vi "Create_Pos_array.vi"(2 "Traverse line":T1 {"Row Duration (mins)" format="%#.1f"; "Row No" min=0; "Trace Gas Concentration (%)" min=0.0 format="%#.2f"; "Emission Rate (l/min)" format="%#.2f"; "Tunnel Speed" format="%#.2f"; "Start X" format="%#.2f"; "Start Y" format="%#.2f"; "Start Z" format="%#.2f"; "End X" format="%#.2f"; "End Y" format="%#.2f"; "End Z" format="%#.2f"; "Averaging time (min)" min=0.0 format="%#.2f"}) -> (5 "Traverse line Out":T1 {"Row Duration (mins)" format="%#.1f"; "Row No" min=0; "Trace Gas Concentration (%)" min=0.0 format="%#.2f"; "Emission Rate (l/min)" format="%#.2f"; "Tunnel Speed" format="%#.2f"; "Start X" format="%#.2f"; "Start Y" format="%#.2f"; "Start Z" format="%#.2f"; "End X" format="%#.2f"; "End Y" format="%#.2f"; "End Z" format="%#.2f"; "Averaging time (min)" min=0.0 format="%#.2f"}, 6 "Error Messages":string, 7 "Array of Positions":dbl[][](array[numeric]) format="%.2f", 9 "Axis Traversed":enum16{"X traverse", "Y traverse", "Z traverse"}(ring))   [LabVIEW 2012]
uses:
  Traverse_cluster.ctl
  Spacing.ctl
  Controls/Multi_run_mode.ctl
  Globals/Extra_Commands_Global.vi
panel:
  # "X           Y            Z"
  # "Start"
  # "End"
  # "X           Y            Z"
  # "Start"
  # "End"
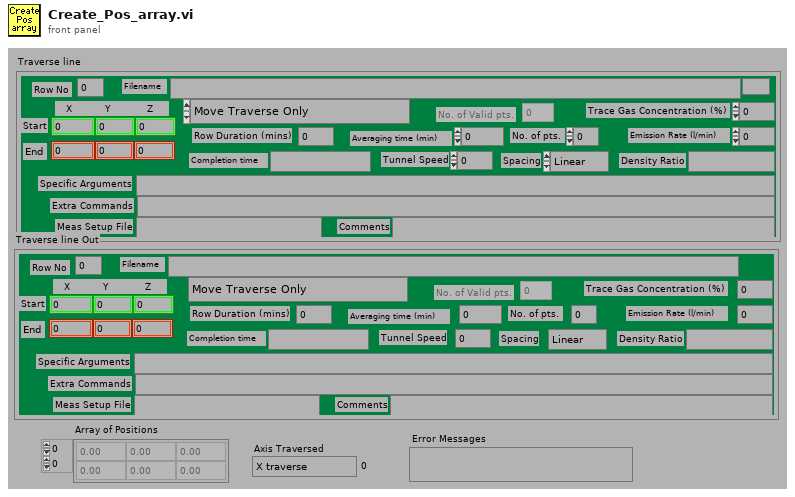
[diagram p1: front panel]
types:
  T1 = typedef "Traverse_cluster.ctl" = cluster{"Start X":dbl, "Start Y":dbl, "Start Z":dbl, "End X":dbl, "End Y":dbl, "End Z":dbl, "No. of pts.":i32, "Spacing":T2, "Filename":path, "Tunnel Speed":dbl, "Averaging time (min)":dbl, "Extra Commands":string, "Specific Arguments":string, "Emission Rate (l/min)":dbl, "Trace Gas Concentration (%)":dbl, "Density Ratio":string, "Comments":string, "Row No":i32, "Row Type Selector":T3, "Completion time":string, "Row Duration (mins)":dbl, "No. of Valid pts.":i32, "Meas Setup File":string}
  T2 = typedef "Spacing.ctl" = enum16{"Linear", "Log", "Gauss", "Specified", "N/A"}
  T3 = typedef "Multi_run_mode.ctl" = enum16{"Move Traverse Only", "Set Tunnel Speed Only", "Set Source Only", "Set Measurement Conditions", "Single Measurement", "Vertical Profile", "Lateral Profile", "Longitudinal Profile", "Explore Volume", "Multi-Axis Profile", "Auto Calibrate", "Meas Fast FID Bkgnd", "Check Beam Power", "Scanning Valve Measurement", "Run VI Named:", "Set ADAM Ch", "Wait (minutes)", "Send Message", "Synchronize With:", "Fall Back to this Row", "Turn Off Row Repeating", "Blank Row", "Traverse 3D Volume"}
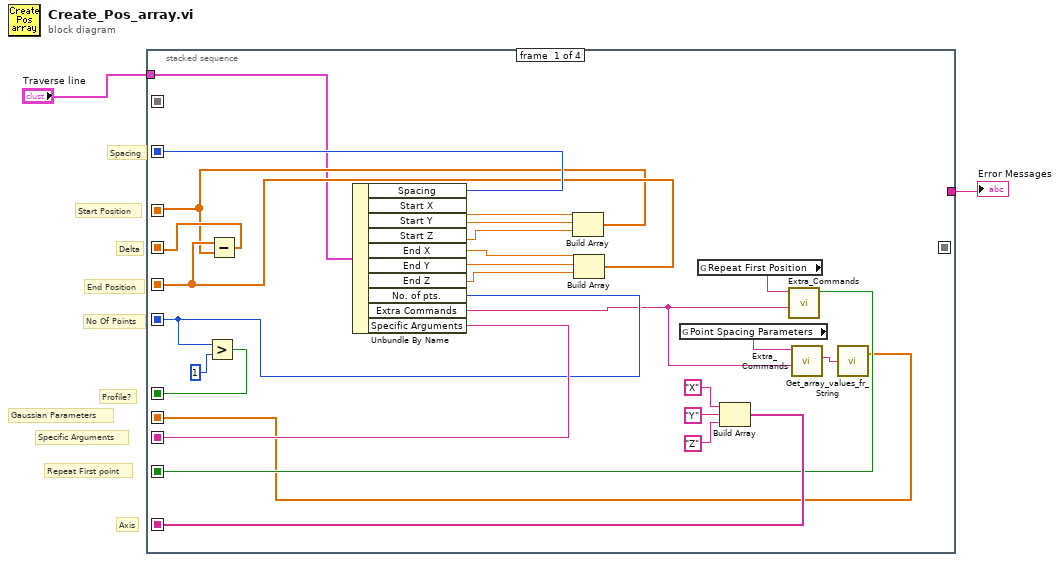
[diagram p0: block diagram]
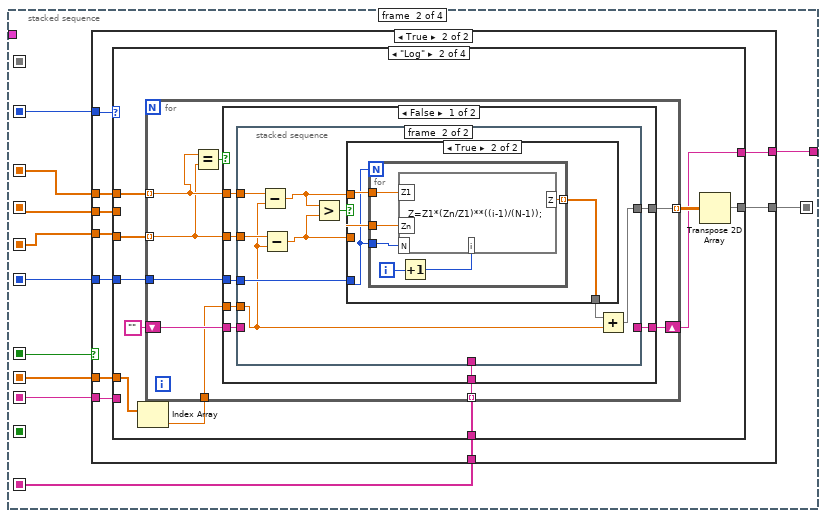
[diagram p2: hidden frame]
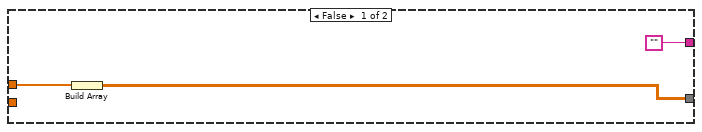
[diagram p3: hidden frame]
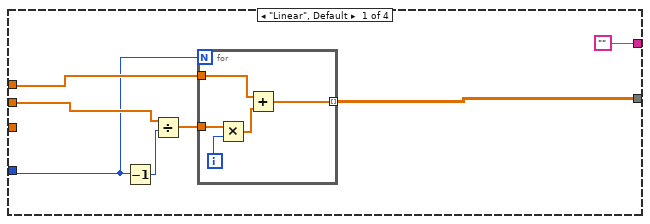
[diagram p4: hidden frame]
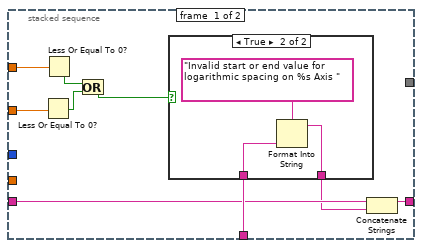
[diagram p5: hidden frame]
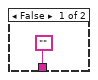
[diagram p6: hidden frame]
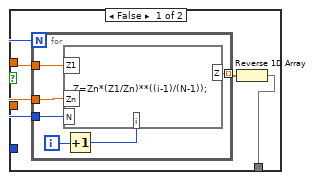
[diagram p7: hidden frame]
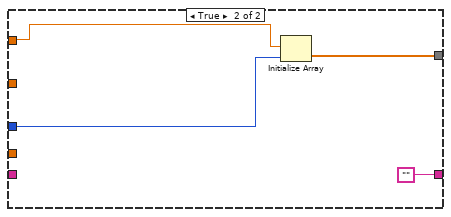
[diagram p8: hidden frame]
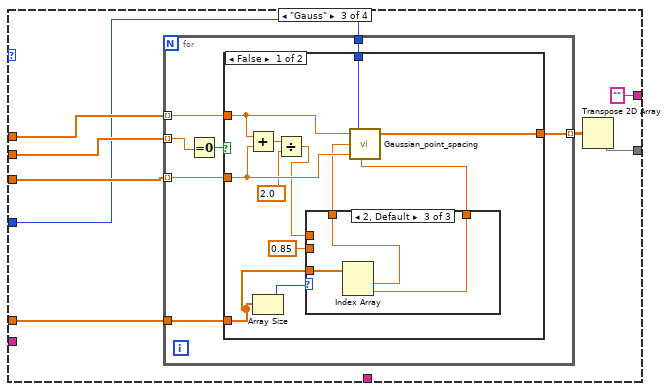
[diagram p9: hidden frame]
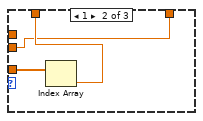
[diagram p11: hidden frame]
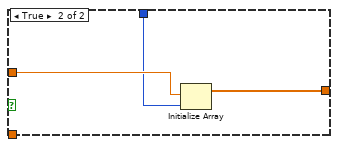
[diagram p12: hidden frame]
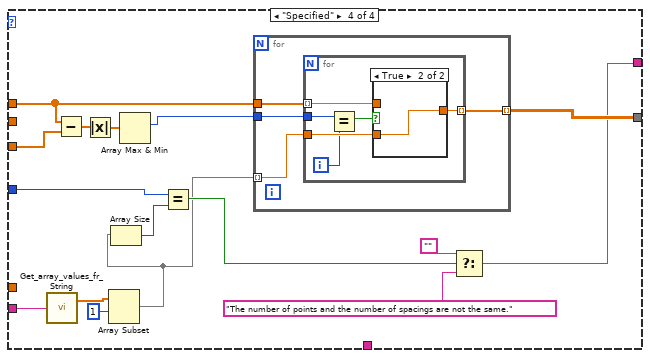
[diagram p13: hidden frame]
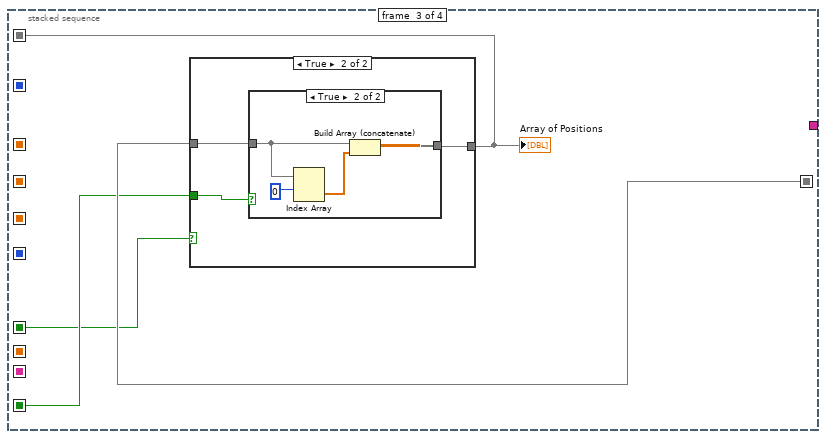
[diagram p15: hidden frame]
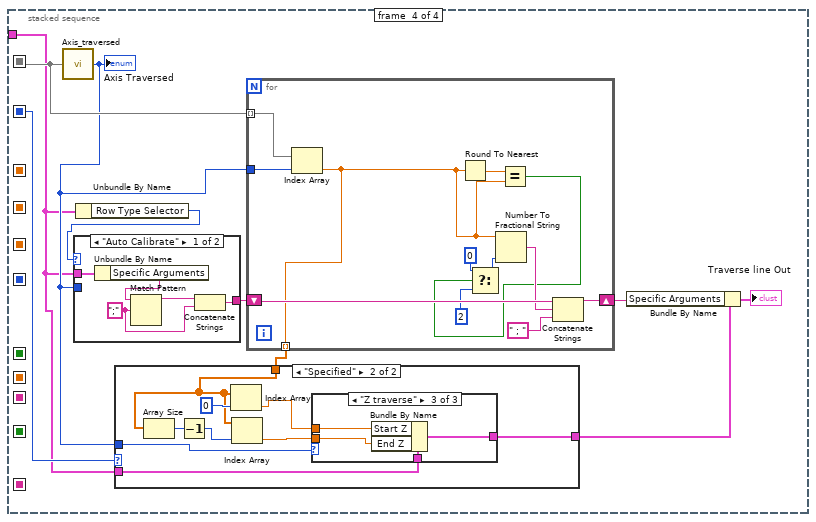
[diagram p18: hidden frame]
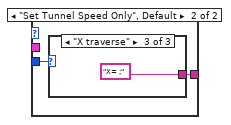
[diagram p19: hidden frame]
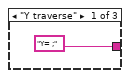
[diagram p20: hidden frame]
diagram:
  # "Gaussian Parameters"
  # "Axis"
  # "Profile?"
  # "Delta"
  # "Repeat First point"
  # "Spacing"
  # "No Of Points"
  # "Specific Arguments"
  # "End Position"
  # "Start Position"
  n1 = stacked-sequence {
    seq-local: [_ w38 _ _] -> [_ _ w207 _]
    seq-local: [w14 _ _ _] -> [_ w35 _ _]
    seq-local: [w19 _ _ _] -> [_ w33 _ _]
    seq-local: [w20 _ _ _] -> [_ w34 _ _]
    seq-local: [w16 _ _ _] -> [_ w31 _ _]
    seq-local: [w18 _ _ _] -> [_ w37 _ _]
    seq-local: [w27 _ _ _] -> [_ w36 _ w222]
    seq-local: [w8 _ _ _] -> [_ _ w206 _]
    seq-local: [w15 _ _ _] -> [_ w30 w205 _]
    seq-local: [w10 _ _ _] -> [_ w29 _ _]
    seq-local: [_ _ w204 _] -> [_ _ _ w226]
    seq-local: [w3 _ _ _] -> [_ w28 _ _]
    tunnel: [_ w32 _ _] -> w2
    tunnel: "Traverse line" -> [w7 _ _ w217]
    frame #0 {
      n2 = Unbundle By Name(w7) -> ("Spacing"=w27:T2, "Start X"=w26:dbl, "Start Y"=w25:dbl, "Start Z"=w24:dbl, "End X"=w23:dbl, "End Y"=w22:dbl, "End Z"=w21:dbl, "No. of pts."=w16:i32, "Extra Commands"=w5:string, "Specific Arguments"=w18:string)
      n3 = Greater?(x=w16, y=1) -> (0:w15:bool)
      n4 = Build Array(w26, w25, w24) -> (w14:dbl[])
      n5 = Build Array(w23, w22, w21) -> (w20:dbl[])
      n6 = Subtract(x=w20, y=w14) -> (x-y=w19:dbl[])
      n7 = global read "Extra_Commands_Global.vi" "Point Spacing Parameters"() -> (w6:string)
      n8 = global read "Extra_Commands_Global.vi" "Repeat First Position"() -> (w9:string)
      n9 = Build Array("X", "Y", "Z") -> (w10:string[])
      n10 = call "Extra_Commands.vi"("String to Search"=w5, "Command"=w9) -> ("Command Found"=w8:bool)  [unwired: 1 in, 4 out]
      n11 = call "Extra_Commands.vi"("String to Search"=w5, "Command"=w6) -> ("String Value"=w4:string)  [unwired: 1 in, 4 out]
      n12 = call "Get_array_values_fr_String.vi"("String Value"=w4) -> ("Numeric Array"=w3:dbl[])  [unwired: 1 out]
    }
    frame #1 {
      n13 = case shown="True" w30 {
        tunnel: [w40 w51] -> w38
        tunnel: w37 -> [_ w50]
        tunnel: w36 -> [_ w49]
        tunnel: w35 -> [w41 w48]
        tunnel: w34 -> [_ w47]
        tunnel: w33 -> [_ w46]
        tunnel: w31 -> [_ w45]
        tunnel: ["" w44] -> w32
        tunnel: w29 -> [_ w43]
        tunnel: w28 -> [_ w42]
        frame False {
          n14 = Build Array(w41) -> (w40:dbl[][])
        }
        frame True {
          n15 = case shown="\"Log\"" w49 {
            tunnel: w47 -> [_ w71 w143 w183]
            tunnel: w48 -> [w57 w72 w144 w179]
            tunnel: w45 -> [w55 w73 w142 w188]
            tunnel: [w58 w70 w141 w190] -> w51
            tunnel: w46 -> [w56 _ w145 _]
            tunnel: w50 -> [_ _ _ w191]
            tunnel: ["" w66 "" ("f") w184] -> w44
            tunnel: w43 -> [_ w68 _ _]
            tunnel: w42 -> [_ w65 w138 _]
            frame "Linear", Default {
              n16 = Decrement(x=w55) -> (x-1=w53:i32)
              n17 = Divide(x=w56, y=w53) -> (x/y=w54:dbl[])
              n18 = for {
                N: w55 -> [_]
                tunnel: w54 -> [w62]
                tunnel: w57 -> [w60]
                tunnel: [w59] -> w58 mode=indexing
                i -> [w63]
                n19 = Multiply(x=w62, y=w63) -> (x*y=w61:dbl[])
                n20 = Add(x=w60, y=w61) -> (x+y=w59:dbl[])
              }
            }
            frame "Log" {
              n21 = Index Array(array=w65) -> (element=w64:dbl)  [unwired: 1 in]
              n22 = for {
                tunnel: [w82] -> w69 mode=indexing
                tunnel: w72 -> [w75] mode=indexing
                tunnel: w71 -> [w74] mode=indexing
                tunnel: w73 -> [w81]
                tunnel: w68 -> [w79] mode=indexing
                shift-right: [w77] -> w66
                shift-left: "" -> [w78]
                tunnel: w64 -> [w76]
                n23 = Equal?(x=w75, y=w74) -> (x = y?=w80:bool)
                n24 = case shown="False" w80 {
                  tunnel: w81 -> [w90 w136]
                  tunnel: w74 -> [w89 _]
                  tunnel: w75 -> [w88 w135]
                  tunnel: [w87 w137] -> w82
                  tunnel: w79 -> [w86 _]
                  tunnel: w78 -> [w85 _]
                  tunnel: [w84 ""] -> w77
                  tunnel: w76 -> [w83 _]
                  frame False {
                    n25 = stacked-sequence {
                      tunnel: [_ w109] -> w87
                      tunnel: w88 -> [w99 w108]
                      tunnel: w89 -> [w98 w107]
                      tunnel: w90 -> [_ w111]
                      tunnel: w86 -> [w94 _]
                      tunnel: w85 -> [w93 _]
                      tunnel: [w91 _] -> w84
                      tunnel: w83 -> [_ w106]
                      frame #0 {
                        n26 = Less Or Equal To 0?(x=w98) -> (x <= 0?=w97:bool)
                        n27 = Less Or Equal To 0?(x=w99) -> (x <= 0?=w96:bool)
                        n28 = Or(x=w96, y=w97) -> (x .or. y?=w95:bool)
                        n29 = case shown="True" w95 {
                          tunnel: w94 -> [_ w103]
                          tunnel: ["" w101] -> w92
                          frame False {
                          }
                          frame True {
                            n30 = Format Into String(format string="Invalid start or end value for logarithmic spacing on %s Axis " ("Format String"), w103) -> (resulting string=w101:string)  [unwired: 2 in, 1 out]
                          }
                        }
                        n31 = Concatenate Strings(w93, w92) -> (w91:string)
                      }
                      frame #1 {
                        n32 = Subtract(x=w108, y=w106) -> (x-y=w104:dbl)
                        n33 = Subtract(x=w107, y=w106) -> (x-y=w105:dbl)
                        n34 = Greater?(x=w104, y=w105) -> (0:w112:bool)
                        n35 = case shown="True" w112 {
                          tunnel: [w114 w124] -> w110
                          tunnel: w104 -> [w113 w127]
                          tunnel: w105 -> [w117 w126]
                          tunnel: w111 -> [w116 w125]
                          frame False {
                            n36 = for {
                              N: w116 -> [_]
                              tunnel: w117 -> [w120]
                              tunnel: w116 -> [w119]
                              tunnel: [w121] -> w115 mode=indexing
                              tunnel: w113 -> [w118]
                              i -> [w123]
                              n37 = Increment(x=w123) -> (x+1=w122:i32)
                              n38 = formula code="Z=Zn*(Z1/Zn)**((i-1)/(N-1));"("i"=w122, "N"=w119, "Zn"=w120, "Z1"=w118) -> ("Z"=w121:dbl)
                            }
                            n39 = Reverse 1D Array(array=w115) -> (reversed array=w114:dbl[])
                          }
                          frame True {
                            n40 = for {
                              N: w125 -> [_]
                              tunnel: w127 -> [w133]
                              tunnel: w126 -> [w132]
                              tunnel: w125 -> [w129]
                              tunnel: [w128] -> w124 mode=indexing
                              i -> [w131]
                              n41 = Increment(x=w131) -> (x+1=w130:i32)
                              n42 = formula code="Z=Z1*(Zn/Z1)**((i-1)/(N-1));"("i"=w130, "N"=w129, "Zn"=w132, "Z1"=w133) -> ("Z"=w128:dbl)
                            }
                          }
                        }
                        n43 = Add(x=w110, y=w106) -> (x+y=w109:dbl[])
                      }
                    }
                  }
                  frame True {
                    n44 = Initialize Array(w135, w136) -> (w137:dbl[])
                  }
                }
              }
              n45 = Transpose 2D Array(2D array=w69) -> (transposed array=w70:dbl[][])
            }
            frame "Gauss" {
              n46 = for {
                tunnel: w145 -> [w147] mode=indexing
                tunnel: w144 -> [w151] mode=indexing
                tunnel: w143 -> [w150] mode=indexing
                tunnel: w142 -> [w149]
                tunnel: [w148] -> w140 mode=indexing
                tunnel: w138 -> [w146]
                n47 = Equal To 0?(x=w147) -> (x = 0?=w152:bool)
                n48 = case shown="False" w152 {
                  tunnel: w151 -> [w162 w175]
                  tunnel: w150 -> [w161 _]
                  tunnel: w149 -> [w164 w174]
                  tunnel: [w163 w173] -> w148
                  tunnel: w146 -> [w154 _]
                  frame False {
                    n49 = Add(x=w162, y=w161) -> (x+y=w160:dbl)
                    n50 = Array Size(array=w154) -> (size(s)=w158:i32)
                    n51 = Divide(x=w160, y=2.0) -> (x/y=w156:dbl)
                    n52 = case shown="2, Default" w158 {
                      tunnel: [w166 w168 w171] -> w157
                      tunnel: w156 -> [w166 _ _]
                      tunnel: [w165 w167 w170] -> w155
                      tunnel: w154 -> [_ w169 w172]
                      tunnel: 0.85 ("Guass intensity") -> [w165 w167 _]
                      frame 0 {
                      }
                      frame 1 {
                        n53 = Index Array(array=w169) -> (element=w168:dbl)  [unwired: 1 in]
                      }
                      frame 2, Default {
                        n54 = Index Array(array=w172) -> (element #1=w171:dbl, element #2=w170:dbl)  [unwired: 2 in]
                      }
                    }
                    n55 = call "Gaussian_point_spacing.vi"("Start point"=w162, "No of points"=w164, "Centre point"=w157, "End point"=w161, "Guass intensity"=w155) -> ("Positions"=w163:dbl[])  [unwired: 2 out]
                  }
                  frame True {
                    n56 = Initialize Array(w175, w174) -> (w173:dbl[])
                  }
                }
              }
              n57 = Transpose 2D Array(2D array=w140) -> (transposed array=w141:dbl[][])
            }
            frame "Specified" {
              n58 = call "Get_array_values_fr_String.vi"("String Value"=w191) -> ("Numeric Array"=w178:dbl[])  [unwired: 1 out]
              n59 = Subtract(x=w179, y=w183) -> (x-y=w182:dbl[])
              n60 = Absolute Value(x=w182) -> (abs(x)=w181:dbl[])
              n61 = Array Subset(array=w178, index=1) -> (w176:dbl[])  [unwired: 1 in]
              n62 = Array Size(array=w176) -> (size(s)=w189:i32)
              n63 = Array Max & Min(array=w181) -> (max index (indices)=w180:i32)  [unwired: 3 out]
              n64 = Equal?(x=w188, y=w189) -> (x = y?=w187:bool)
              n65 = for {
                tunnel: w176 -> [w193] mode=indexing
                tunnel: [w194] -> w190 mode=indexing
                tunnel: w180 -> [w195]
                tunnel: w179 -> [w192]
                n66 = for {
                  tunnel: w195 -> [w199]
                  tunnel: [w201] -> w194 mode=indexing
                  tunnel: w193 -> [w200]
                  tunnel: w192 -> [w196] mode=indexing
                  i -> [w198]
                  n67 = Equal?(x=w199, y=w198) -> (x = y?=w197:bool)
                  n68 = case shown="True" w197 {
                    tunnel: [w202 w203] -> w201
                    tunnel: w200 -> [_ w203]
                    tunnel: w196 -> [w202 _]
                    frame False {
                    }
                    frame True {
                    }
                  }
                }
              }
              n69 = Select(t="", s=w187, f="The number of points and the number of spacings are not the same.") -> (s? t:f=w184:string)
            }
          }
        }
      }
    }
    frame #2 {
      n70 = case shown="True" w205 {
        tunnel: [w208 w211] -> w204
        tunnel: w207 -> [w208 w210]
        tunnel: w206 -> [_ w209]
        frame False {
        }
        frame True {
          n71 = case shown="True" w209 {
            tunnel: [w212 w216] -> w211
            tunnel: w210 -> [w212 w214]
            frame False {
            }
            frame True {
              n72 = Index Array(array=w214, index (row)=0) -> (element=w215:dbl[])  [unwired: 1 in]
              n73 = Build Array (concatenate)(w214, w215) -> (w216:dbl[][])
            }
          }
        }
      }
      "Array of Positions" <- w204
    }
    frame #3 {
      n74 = call "Axis_traversed.vi"("Position array"=w226) -> ("Axis Traversed"=w220:enum16{"X traverse", "Y traverse", "Z traverse"})  [unwired: 4 out]
      "Axis Traversed" <- w220
      n75 = Unbundle By Name(w217) -> ("Row Type Selector"=w218:T3)
      n76 = case shown="\"Auto Calibrate\"" w218 {
        tunnel: [w229 w233] -> w223
        tunnel: w220 -> [_ w232]
        tunnel: w217 -> [w231 _]
        frame "Auto Calibrate" {
          w227 = ";" ("regular expression")
          n77 = Unbundle By Name(w231) -> ("Specific Arguments"=w230:string)
          n78 = Match Pattern(string=w230, regular expression=w227) -> (before substring=w228:string)  [unwired: 4 out]
          n79 = Concatenate Strings(w228, w227) -> (w229:string)
        }
        frame "Set Tunnel Speed Only", Default {
          n80 = case shown="\"X traverse\"" w232 {
            tunnel: ["Y= ;" "Z= ;" "X= ;"] -> w233
            frame "Y traverse" {
            }
            frame "Z traverse" {
            }
            frame "X traverse" {
            }
          }
        }
      }
      n81 = for {
        tunnel: w220 -> [w270]
        tunnel: w226 -> [w260] mode=indexing
        shift-right: [w268] -> w225
        shift-left: w223 -> [w269]
        tunnel: [w259] -> w221 mode=indexing
        n82 = Index Array(array=w260, index=w270) -> (element=w259:dbl)
        n83 = Round To Nearest(number=w259) -> (nearest integer value=w262:dbl)
        n84 = Equal?(x=w262, y=w259) -> (x = y?=w261:bool)
        n85 = Select(t=0, s=w261, f=2) -> (s? t:f=w265:i32)
        n86 = Number To Fractional String(number=w259, precision (6)=w265) -> (F-format string=w267:string)  [unwired: 2 out]
        n87 = Concatenate Strings(w269, w267, " ; " ("string")) -> (w268:string)
      }
      n88 = case shown="\"Specified\"" w222 {
        tunnel: w221 -> [_ w241]
        tunnel: w220 -> [_ w246]
        tunnel: w217 -> [w237 w245]
        tunnel: [w237 w240] -> w219
        frame "Linear", Default {
        }
        frame "Specified" {
          n89 = Array Size(array=w241) -> (size(s)=w244:i32)
          n90 = Decrement(x=w244) -> (x-1=w242:i32)
          n91 = Index Array(array=w241, index=0) -> (element=w239:dbl)
          n92 = Index Array(array=w241, index=w242) -> (element=w238:dbl)
          n93 = case shown="\"Z traverse\"" w246 {
            tunnel: w245 -> [w250 w254 w258]
            tunnel: [w249 w253 w257] -> w240
            tunnel: w239 -> [w248 w252 w256]
            tunnel: w238 -> [w247 w251 w255]
            frame "X traverse" {
              n94 = Bundle By Name(cluster=w250, "Start X"=w248, "End X"=w247) -> (w249:T1)
            }
            frame "Y traverse" {
              n95 = Bundle By Name(cluster=w254, "Start Y"=w252, "End Y"=w251) -> (w253:T1)
            }
            frame "Z traverse" {
              n96 = Bundle By Name(cluster=w258, "Start Z"=w256, "End Z"=w255) -> (w257:T1)
            }
          }
        }
      }
      n97 = Bundle By Name(cluster=w219, "Specific Arguments"=w225) -> (→"Traverse line Out":T1)
    }
  }
  "Error Messages" <- w2
